vi "MotorsGlobal.vi"() -> ()   [LabVIEW 2019]
uses:
  TurretMode.ctl
panel:
  out "Amount of balls":dbl
  in  "IR1":bool
  in  "IR0":bool
  in  "TurretMode":T1
  in  "AutoTurret":bool
  in  "RollerOutput":dbl
  in  "ClimberSolenoid":bool
  in  "HoodSolenoid":bool
  in  "IntakeSolenoid":bool
  out "LimelightY":dbl
  out "LimelightX":dbl
  out "FlyWheelRate":dbl
  out "FlyWheelEncoder":dbl
  in  "ConveyorRightOutput":dbl
  in  "ConveyorLeftOutput":dbl
  in  "ConveyorMidOutput":dbl
  in  "IntakeOutput":dbl
  in  "TurretOutput":dbl
  in  "FlywheelOutput":dbl
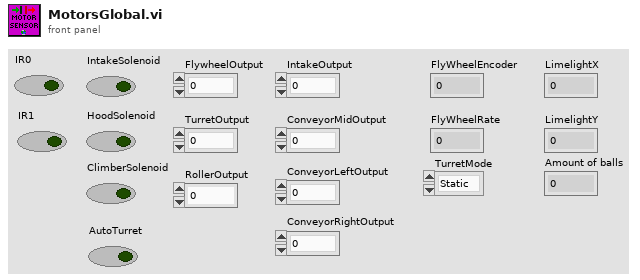
[diagram p1: front panel]
types:
  T1 = typedef "TurretMode.ctl" = enum16{"Static", "Manual", "Automatic"}
diagram:
